vi "popularVideos.vi"(8 "error in (no error)":errorcluster, 11 "ThirdPartyYoutubeClass in":refnum<class "ThirdPartyYoutubeClass.lvclass">) -> (0 "error out":errorcluster, 2 "HashMap":T1, 3 "ThirdPartyYoutubeClass out":refnum<class "ThirdPartyYoutubeClass.lvclass">)   [LabVIEW 2017, in "ThirdPartyYoutubeClass.lvclass"]
uses:
  ThirdPartyYoutubeClass.lvclass
  Video Class/Video.lvclass
  ThirdPartyYoutubeLib Class/ThirdPartyYoutubeLib.lvclass
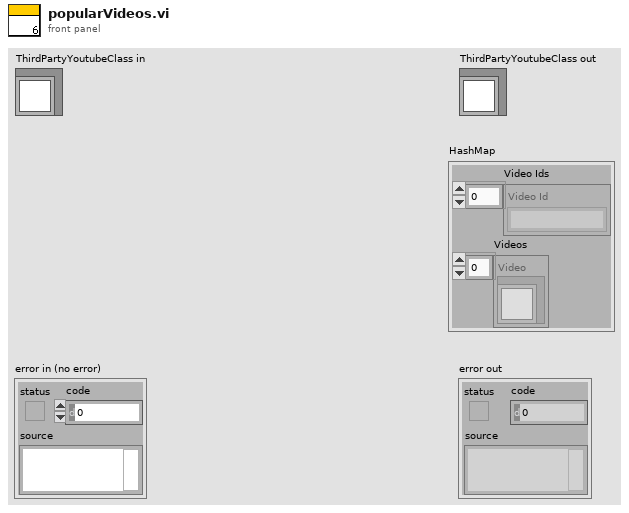
[diagram p1: front panel]
types:
  T1 = cluster{"Video Ids":string[], "Videos":refnum<class "Video.lvclass">[]}
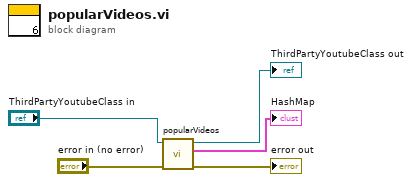
[diagram p0: block diagram]
diagram:
  n1 = call-parent "popularVideos.vi"("error in (no error)"="error in (no error)", "ThirdPartyYoutubeLib in"="ThirdPartyYoutubeClass in") -> ("error out"=→"error out":errorcluster, "HashMap"=→"HashMap":T1, "ThirdPartyYoutubeLib out"=→"ThirdPartyYoutubeClass out":refnum<class "ThirdPartyYoutubeClass.lvclass">)  [unwired: 7 in]
